vi "Forward.vi"(8 "error in":errorcluster, 11 "Tree":refnum<vi>) -> (0 "error out":errorcluster)   [LabVIEW 2020]
uses:
  <vilib>/Utility/miscctls.llb/LVNodeAndColumnTypeDef.ctl
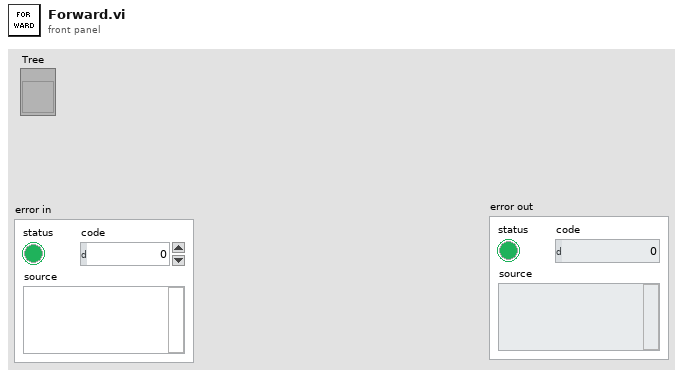
[diagram p1: front panel]
types:
  T1 = typedef "LVNodeAndColumnTypeDef.ctl" = cluster{"Node":string, "Column":i32}
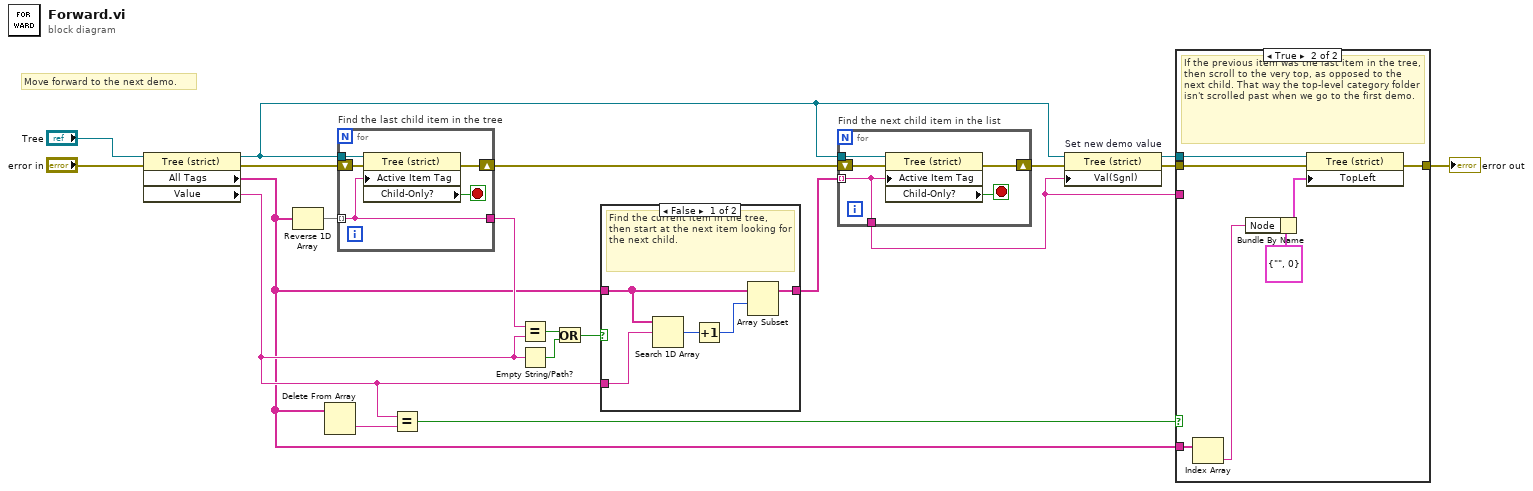
[diagram p0: block diagram]
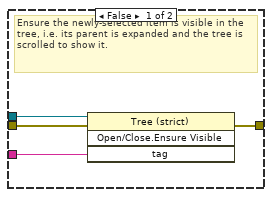
[diagram p2: hidden frame]
diagram:
  # "Move forward to the next demo."
  n1 = property class="Tree (strict)"(reference="Tree", error in="error in") -> (reference out=w11:refnum<vi>, error out=w13:errorcluster, "All Tags"=w1:string[], "Value"=w3:string)
  n2 = Reverse 1D Array(array=w1) -> (reversed array=w9:string[])
  n3 = Delete From Array(array=w1) -> (deleted portion=w4:string)  [unwired: 2 in, 1 out]
  n4 = for "Find the last child item in the tree" {
    shift-right: [w24] -> w12
    shift-left: w13 -> [w25]
    tunnel: w11 -> [w23]
    tunnel: w9 -> [w22] mode=indexing
    tunnel: [w22] -> w10
    stop <- w21 stop-if-true
    n5 = property class="Tree (strict)"(reference=w23, error in=w25, "Active Item Tag"=w22) -> (error out=w24:errorcluster, "Child-Only?"=w21:bool)  [unwired: 1 out]
  }
  n6 = Equal?(x=w3, y=w4) -> (x = y?=w2:bool)
  n7 = Equal?(x=w10, y=w3) -> (x = y?=w17:bool)
  n8 = Empty String/Path?(string/path=w3) -> (empty?=w16:bool)
  n9 = Or(x=w17, y=w16) -> (x .or. y?=w15:bool)
  n10 = case shown="False" w15 {
    tunnel: w1 -> [w29 w31]
    tunnel: w3 -> [w30 _]
    tunnel: [w26 w31] -> w14
    frame False {
      # "Find the current item in the tree, then start at the next item looking for the next child."
      n11 = Search 1D Array(1D array=w29, element=w30) -> (index of element=w28:i32)  [unwired: 1 in]
      n12 = Increment(x=w28) -> (x+1=w27:i32)
      n13 = Array Subset(array=w29, index=w27) -> (w26:string[])  [unwired: 1 in]
    }
    frame True {
      # "If there is no item selected in the tree (or the last child item is selected), then find the first child item in the tree."
    }
  }
  n14 = for "Find the next child item in the list" {
    shift-right: [w35] -> w19
    shift-left: w12 -> [w36]
    tunnel: w11 -> [w34]
    tunnel: w14 -> [w32] mode=indexing
    tunnel: [w32] -> w6
    stop <- w33 stop-if-true
    n15 = property class="Tree (strict)"(reference=w34, error in=w36, "Active Item Tag"=w32) -> (error out=w35:errorcluster, "Child-Only?"=w33:bool)  [unwired: 1 out]
  }
  n16 = property on="Set new demo value" class="Tree (strict)"(reference=w11, error in=w19, "Val(Sgnl)"=w6) -> (reference out=w8:refnum<vi>, error out=w7:errorcluster)
  n17 = case shown="True" w2 {
    tunnel: w8 -> [w40 w45]
    tunnel: w7 -> [w39 w46]
    tunnel: w6 -> [w38 _]
    tunnel: [w37 w47] -> w5
    tunnel: w1 -> [_ w42]
    frame False {
      # "Ensure the newly-selected item is visible in the tree, i.e. its parent is expanded and the tree is scrolled to show it."
      n18 = invoke class="Tree (strict)" method="Open/Close.Ensure Visible"(reference=w40, error in=w39, "tag"=w38) -> (error out=w37:errorcluster)  [unwired: 1 in, 3 out]
    }
    frame True {
      # "If the previous item was the last item in the tree, then scroll to the very top, as opposed to the next child. That way the top-level category folder isn't scrolled past when we go to the first demo."
      n19 = Index Array(array=w42) -> (element=w41:string)  [unwired: 1 in]
      n20 = Bundle By Name(cluster=T1 {"Node"="", "Column"=0} ("Top Left Visible Cell"), "Node"=w41) -> (w43:T1)
      n21 = property class="Tree (strict)"(reference=w45, error in=w46, "TopLeft"=w43) -> (error out=w47:errorcluster)  [unwired: 1 out]
    }
  }
  "error out" <- w5
